vi "moveHEV01-02.vi"(8 "error in":errorcluster, 10 "IndexFlow":i32) -> (0 "error out 2":errorcluster caption="error out")   [LabVIEW 2012]
uses:
  GlobalVariables/GantnerParameters.vi
  GlobalVariables/CommunicationActivity.vi
  ISMBUS32.DLL
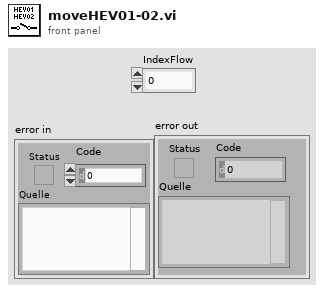
[diagram p1: front panel]
types:
  T1 = typedef "ISMBUS_Module.ctl" = cluster{"ModuleAddress":i32, "ModuleKindIndex":i32, "ModuleKind":string, " Protocol":string, " BaudRate":i32, "CharFormat":string, "BaudRateIndex":i32, "FormatIndex":i32, "ProtocolIndex":i32, "Location":string, "SerialNumber":string, "Vendor":string, "HWRelease":string, "SWRelease":string, "ControllerType":string, "ChannelList":T2[], "ChannelCount":i32, " COM Port":i32}
  T2 = typedef "ISMBUS_Channel.ctl" = cluster{" Description":string, " ChannelKindIndex":i32, "ChannelFormatIndex":i32, " FieldLength":i32, "Precision":i32, "Unit":string, "Mode":i32}
  T3 = cluster{"Module":T1, "PT01 chanel":u32, "Temperature chanel":u32, "HEV01 chanel":u32, "HEV02 chanel":u32, "PressureLimit":dbl}
  T4 = cluster{"KellerActive":bool, "GantnerActive":bool, "BrooksActive":bool}
  T5 = cluster{"KellerActive":bool, bool, "BrooksActive":bool}
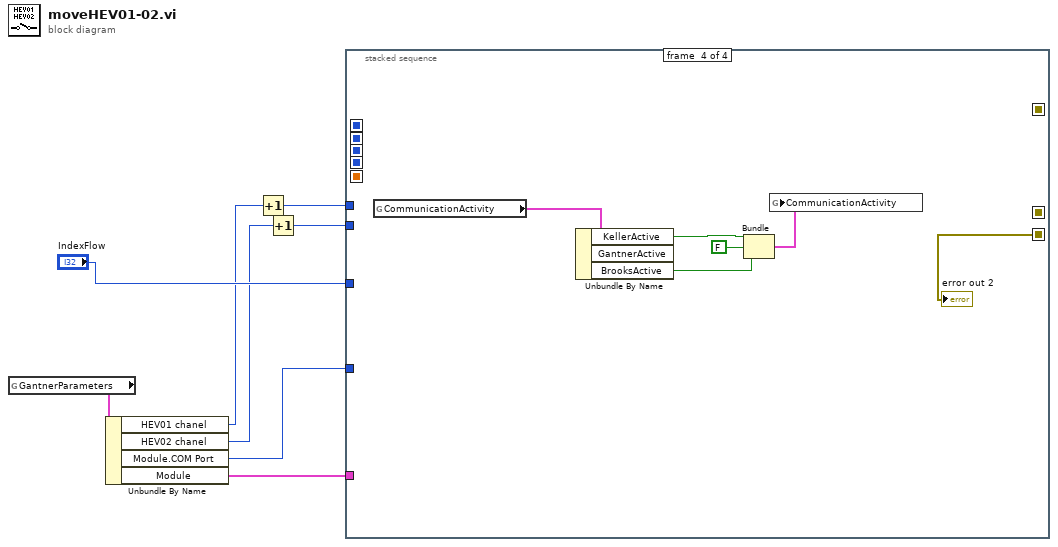
[diagram p0: block diagram]
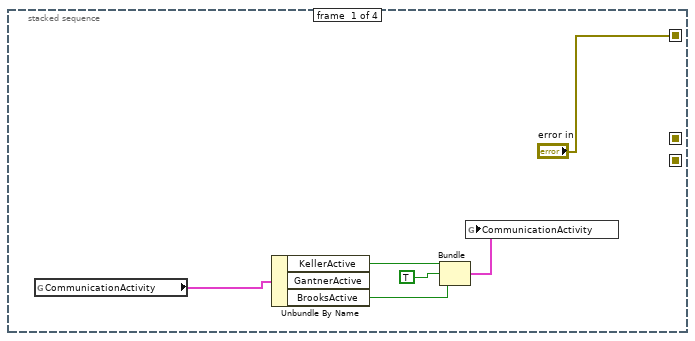
[diagram p2: hidden frame]
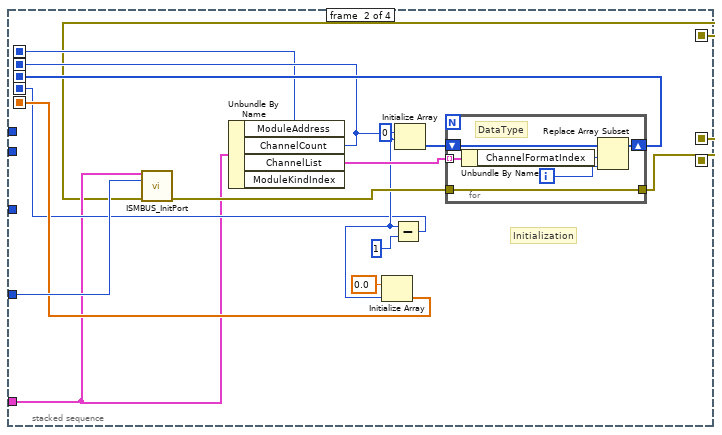
[diagram p3: hidden frame]
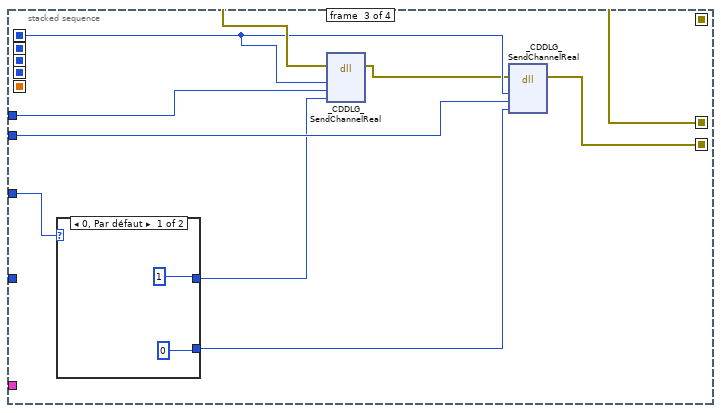
[diagram p4: hidden frame]
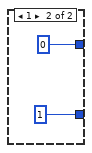
[diagram p5: hidden frame]
diagram:
  n1 = global read "GantnerParameters.vi" "GantnerParameters"() -> (w8:T3)
  n2 = Unbundle By Name(w8) -> ("HEV01 chanel"=w1:u32, "HEV02 chanel"=w3:u32, "Module.COM Port"=w7:i32, "Module"=w6:T1)
  n3 = Increment(x=w1) -> (x+1=w2:u32)
  n4 = Increment(x=w3) -> (x+1=w4:u32)
  n5 = stacked-sequence {
    seq-local: [_ w17 _ _] -> [_ _ w41 _]
    seq-local: [_ w20 _ _] -> [_ _ _ _]
    seq-local: [_ w22 _ _] -> [_ _ _ _]
    seq-local: [_ w19 _ _] -> [_ _ _ _]
    seq-local: [_ w21 _ _] -> [_ _ _ _]
    seq-local: ["error in" _ _ _] -> [_ w16 _ _]
    seq-local: [_ w15 _ _] -> [_ _ w43 _]
    seq-local: [_ _ w39 _] -> [_ _ _ w51]
    tunnel: w7 -> [_ w29 _ _]
    tunnel: w6 -> [_ w18 _ _]
    tunnel: w2 -> [_ _ w44 _]
    tunnel: w4 -> [_ _ w42 _]
    tunnel: "IndexFlow" -> [_ _ w36 _]
    frame #0 {
      n6 = global read "CommunicationActivity.vi" "CommunicationActivity"() -> (w14:T4)
      n7 = Unbundle By Name(w14) -> ("KellerActive"=w10:bool, "BrooksActive"=w12:bool)  [unwired: 1 out]
      n8 = Bundle("KellerActive"=w10, TRUE, "BrooksActive"=w12) -> (w13:T5)  [unwired: 1 in]
      n9 = global write "CommunicationActivity.vi" "CommunicationActivity"(w13) -> ()
    }
    frame #1 {
      # "Initialization"
      n10 = call "ISMBUS_InitPort.vi"("Module"=w18, "ComPort"=w29, "Fehler (Eingang - kein Fehler)"=w16) -> ("Fehler (Ausgang)"=w23:errorcluster)  [unwired: 12 out]
      n11 = Unbundle By Name(w18) -> ("ModuleAddress"=w17:i32, "ChannelCount"=w20:i32, "ChannelList"=w26:T2[])  [unwired: 1 out]
      n12 = Initialize Array(0.0, w20) -> (w21:dbl[])
      n13 = Subtract(x=w20, y=1) -> (x-y=w19:i32)
      n14 = Initialize Array(0 ("Element"), w20) -> (w27:i32[])
      n15 = for {
        tunnel: w26 -> [w34] mode=indexing
        shift-right: [w32] -> w22
        shift-left: w27 -> [w31]
        tunnel: w23 -> [w30]
        tunnel: [w30] -> w15
        i -> [w35]
        # "DataType"
        n16 = Unbundle By Name(w34) -> ("ChannelFormatIndex"=w33:i32)
        n17 = Replace Array Subset(array=w31, new element=w33, index=w35) -> (w32:i32[])
      }
    }
    frame #2 {
      n18 = case shown="0, Par défaut" w36 {
        tunnel: [1 0] -> w38
        tunnel: [0 1] -> w37
        frame 0, Default {
        }
        frame 1 {
        }
      }
      n19 = dll-call lib="ISMBUS32.DLL" fn="_CDDLG_SendChannelReal"(error in=w43, "Address"=w41, "NumCh"=w44, "Value"=w38) -> (error out=w40:errorcluster)  [unwired: 5 in, 2 out]
      n20 = dll-call lib="ISMBUS32.DLL" fn="_CDDLG_SendChannelReal"(error in=w40, "Address"=w41, "NumCh"=w42, "Value"=w37) -> (error out=w39:errorcluster)  [unwired: 5 in, 2 out]
    }
    frame #3 {
      n21 = global read "CommunicationActivity.vi" "CommunicationActivity"() -> (w54:T4)
      n22 = Unbundle By Name(w54) -> ("KellerActive"=w50:bool, "BrooksActive"=w52:bool)  [unwired: 1 out]
      n23 = Bundle("KellerActive"=w50, FALSE, "BrooksActive"=w52) -> (w53:T5)  [unwired: 1 in]
      n24 = global write "CommunicationActivity.vi" "CommunicationActivity"(w53) -> ()
      "error out 2" <- w51
    }
  }
